vi "test_SessionsReserved_ReserveSessions_ReturnsError.vi"(8 "error in":errorcluster) -> (0 "error out":errorcluster, 2 "result":string, 3 "pass":bool)   [LabVIEW 2020, in "MeasurementServerTests.lvlib" / "Session Reservation Tests.lvlib"]
uses:
  Session Reservation Tests.lvlib
  MeasurementServerTests.lvlib
  Runtime/Clients/Session Management V1/Session Reservation/Session Reservation.lvclass
  gRPC/Generated APIs/ni/measurementlink/sessionmanagement/v1/RPC Messages/ni_measurementlink_PinMapContext.ctl
  gRPC/Generated APIs/ni/measurementlink/sessionmanagement/v1/ni.measurementlink.sessionmanagement.v1.api.lvlib
  Helpers/Pin Map XML Strings Global.vi
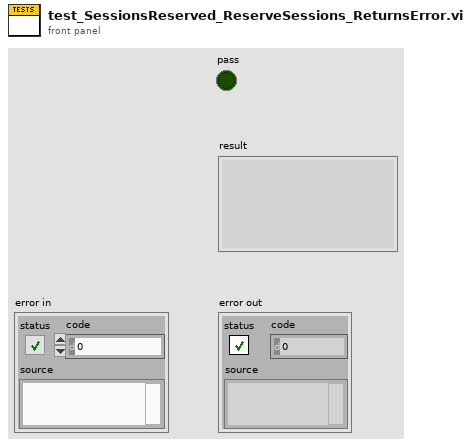
[diagram p1: front panel]
types:
  T1 = typedef "ni.measurementlink.sessionmanagement.v1.api.lvlib/ni_measurementlink_PinMapContext.ctl" = cluster{"pin_map_id":string, "sites":i32[]}
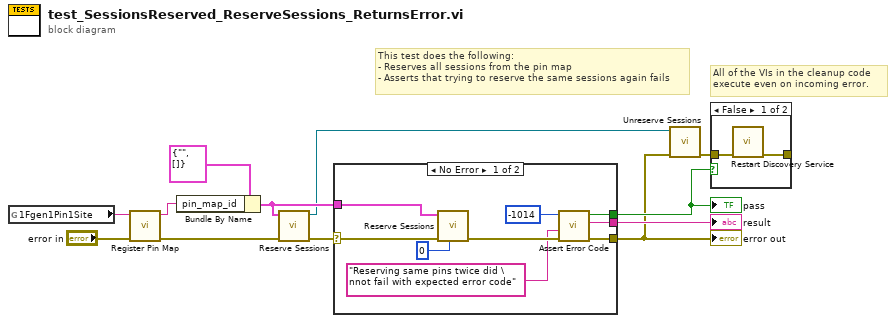
[diagram p0: block diagram]
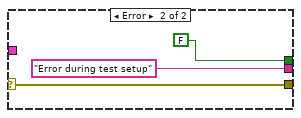
[diagram p2: hidden frame]
diagram:
  # "All of the VIs in the cleanup code\nexecute even on incoming error."
  # "This test does the following:\n- Reserves all sessions from the pin map\n- Asserts that trying to reserve the same sessions again fails"
  n1 = global read "Pin Map XML Strings Global.vi" "1Fgen1Pin1Site"() -> (w6:string)
  n2 = call "Register Pin Map.vi"("error in"="error in", "pin map xml"=w6) -> ("error out"=w9:errorcluster, "pin map id"=w7:string)  [unwired: 8 in]
  n3 = Bundle By Name(cluster=T1 {"pin_map_id"="", "sites"=[]} ("pin map context"), "pin_map_id"=w7) -> (w3:T1)
  n4 = call "Reserve Sessions.vi"("error in"=w9, "pin map context"=w3) -> ("error out"=w4:errorcluster, "session reservation out"=w1:refnum<class "Session Reservation.lvclass">)  [unwired: 8 in]
  n5 = case shown="No Error" w4 {
    selector: w4 -> [w18 w22]
    tunnel: [w13 w22] -> w10
    tunnel: [w15 FALSE] -> w11
    tunnel: [w14 "Error during test setup" ("f")] -> w12
    tunnel: w3 -> [w16 _]
    frame No Error {
      n6 = call "Reserve Sessions.vi"("timeout (ms)"=0, "error in"=w18, "pin map context"=w16) -> ("error out"=w21:errorcluster)  [unwired: 7 in, 1 out]
      n7 = call "Assert Error Code.vi"("error in"=w21, "additional info to prepend"="Reserving same pins twice did \nnot fail with expected error code", "expected error code"=-1014) -> ("error out"=w13:errorcluster, "details"=w14:string, "error code match?"=w15:bool)  [unwired: 6 in]
    }
    frame Error {
    }
  }
  "error out" <- w10
  "pass" <- w11
  "result" <- w12
  n8 = call "Unreserve Sessions.vi"("error in"=w10, "session reservation in"=w1) -> ("error out"=w2:errorcluster)  [unwired: 9 in]
  n9 = case shown="False" w11 {
    tunnel: w2 -> [w26 _]
    tunnel: [w25 _] -> _
    frame False {
      n10 = call "Restart Discovery Service.vi"("error in"=w26) -> ("error out"=w25:errorcluster)  [unwired: 10 in]
    }
    frame True {
    }
  }
